vi "test_connector_Raise Error for Sets Before 2024.vi"(8 "error in (no error)":errorcluster) -> (0 "error out":errorcluster, 2 "supported?":bool)   [LabVIEW 2020, in "openg_variant.lvlib"]
uses:
  openg_variant.lvlib
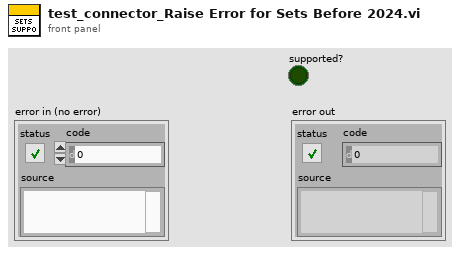
[diagram p1: front panel]
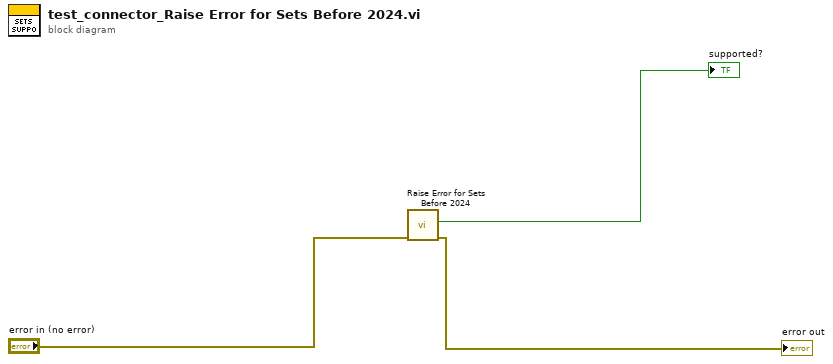
[diagram p0: block diagram]
diagram:
  n1 = call "Raise Error for Sets Before 2024.vi"("error in (no error)"="error in (no error)") -> ("error out"=→"error out":errorcluster, "supported?"=→"supported?":bool)  [unwired: 9 in]
